vi "FetchSpecificationDataFromDb.vi"() -> ()   [LabVIEW 2019]
uses:
  <vilib>/addons/database/Auxilliary.llb/DB Tools Parameter Info.ctl
  <vilib>/addons/database/Auxilliary.llb/DB Tools DataTypes.ctl
  <vilib>/addons/database/Auxilliary.llb/DB Tools Parameter Dir.ctl
  <vilib>/addons/database/Auxilliary.llb/DB Tools Format Datetime String (Time Stamp).vi
  <vilib>/addons/database/Connection.llb/DB Tools Open Connec (String).vi
  <vilib>/addons/database/Command.llb/Cmd Set Parameter Value (C).vi
  <vilib>/addons/database/Command.llb/Cmd Execute.vi
  <vilib>/addons/database/Recordset.llb/Rec Fetch Recordset Data (CR).vi
  <vilib>/addons/database/Recordset.llb/Rec Destroy - Command.vi
  <vilib>/addons/database/Command.llb/Cmd Delete.vi
  <vilib>/addons/database/Recordset.llb/Rec Fetch String Data (CR).vi
  <vilib>/addons/database/NI_Database_API.lvlib
panel:
  out "tables":string[](array[string])
  out "data":string
  out "Program end (seconds)":dbl
  out "Programe fetched data time":timestamp
  out "Programme start time":timestamp
  out "size(s)":i32[](array[numeric])
  in  "Provide your To DateTime here":timestamp
  in  "Provide your from  DateTime here":timestamp
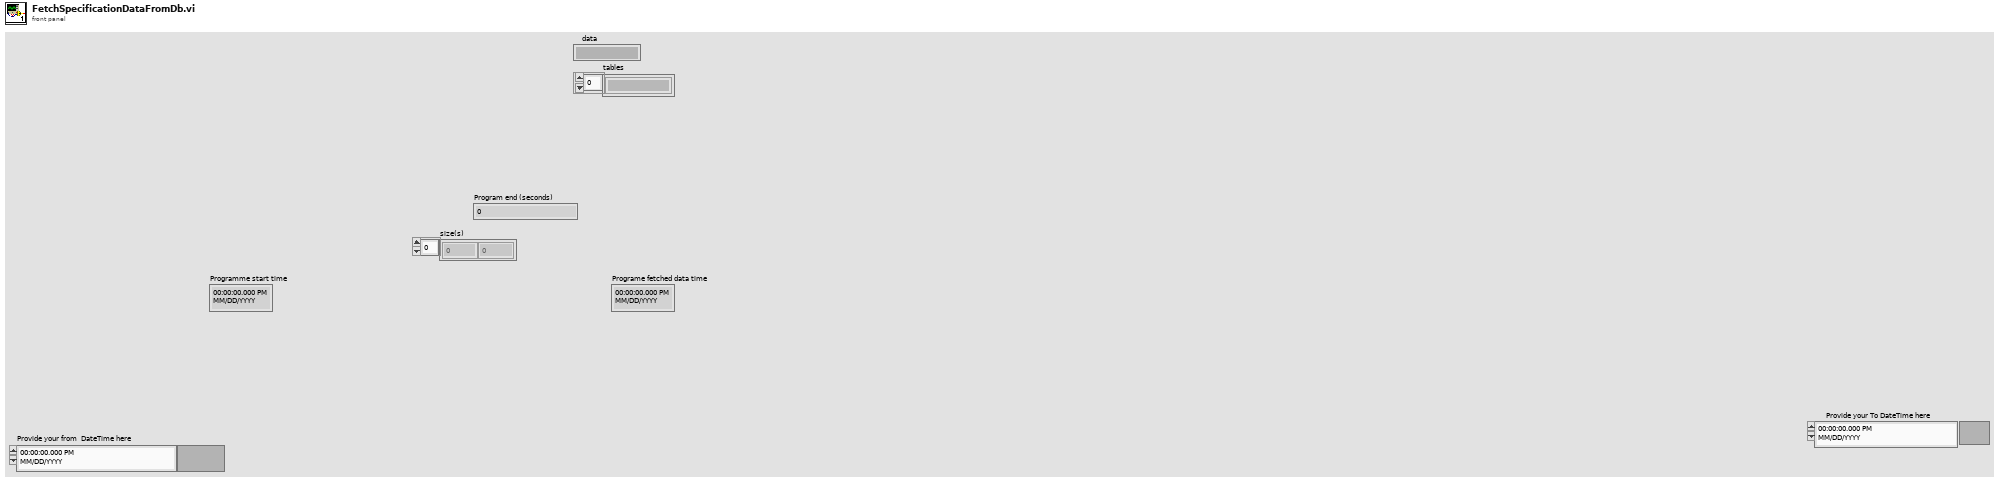
[diagram p1: front panel]
types:
  T1 = typedef "NI_Database_API.lvlib/DB Tools Parameter Info.ctl" = cluster{"parameter name":string, "type":T2, "direction":T3, "value":variant}
  T2 = typedef "NI_Database_API.lvlib/DB Tools DataTypes.ctl" = enum16{"String", "Long (I32)", "Single (SGL)", "Double (DBL)", "Date/Time", "Binary"}
  T3 = typedef "NI_Database_API.lvlib/DB Tools Parameter Dir.ctl" = enum32{"Input", "Output", "Input/Output", "Return Value"}
  T4 = typedef "NI_Database_API.lvlib/Conn ObjectReference.ctl" = refnum<k1>
  T5 = typedef "NI_Database_API.lvlib/Cmd ObjectReference.ctl" = refnum<k1>
  T6 = typedef "NI_Database_API.lvlib/Cmd-Rec Object Reference.ctl" = refnum<k1>
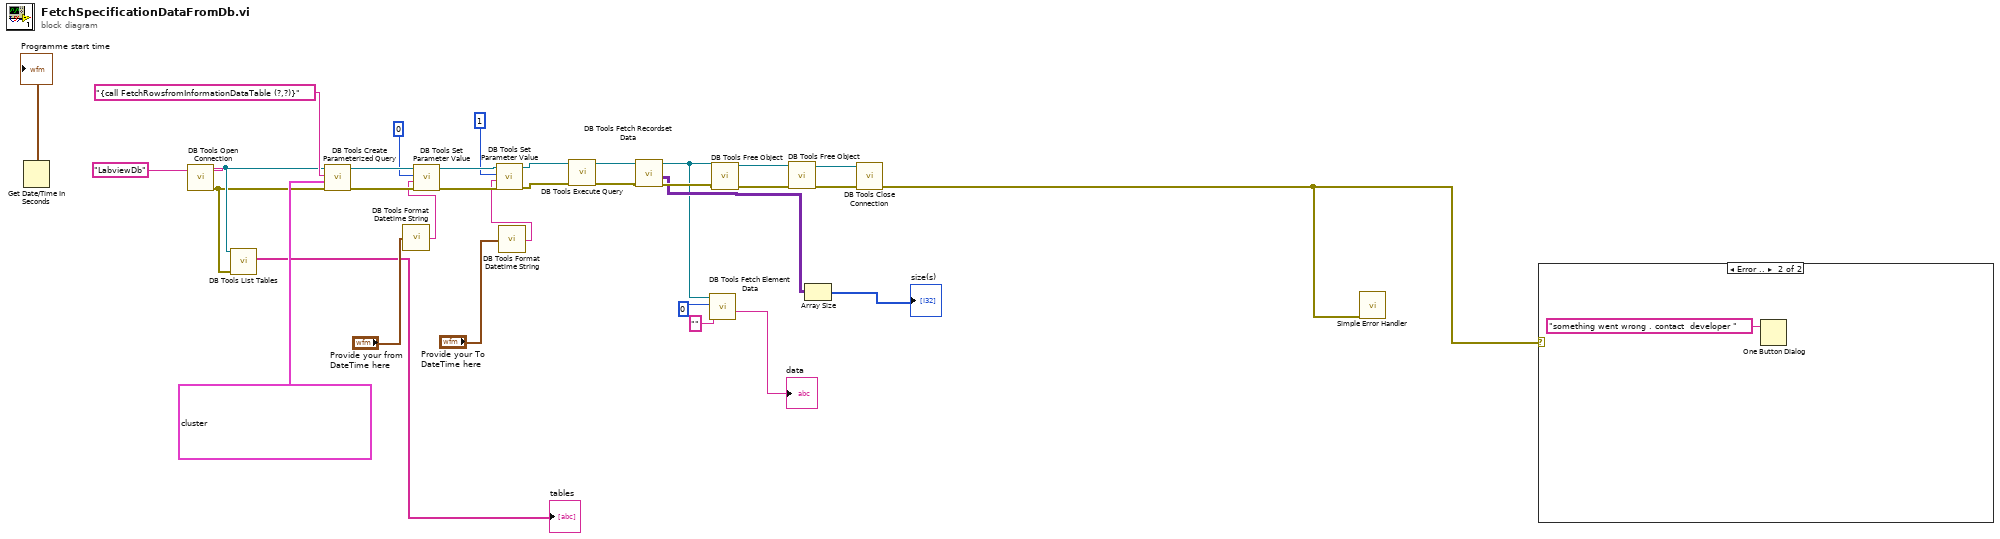
[diagram p0: block diagram]
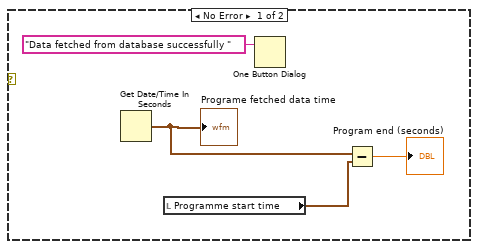
[diagram p2: hidden frame]
diagram:
  n1 = Get Date/Time In Seconds() -> (seconds since 1Jan1904=→"Programme start time":timestamp)
  n2 = call-poly <vilib>:"DB Tools Open Connection.vi"("connection information"="LabviewDb") -> ("error out"=w2:errorcluster, "connection reference"=w3:T4)  [unwired: 7 in]
  n3 = call <vilib>:"DB Tools List Tables.vi"("error in (no error)"=w2, "connection reference"=w3) -> ("tables"=→"tables":string[])  [unwired: 3 in, 2 out]
  n4 = call <vilib>:"DB Tools Create Parameterized Query.vi"("error in (no error)"=w2, "parameters"=T1[] [{"parameter name"="fromDate", "type"=enum."Date/Time", "direction"=enum."Input", "value"=variant}, {"parameter name"="toDate", "type"=enum."Date/Time", "direction"=enum."Input", "value"=variant}], "SQL query"="{call FetchRowsfromInformationDataTable (?,?)}", "connection reference"=w3) -> ("error out"=w30:errorcluster, "command reference"=w29:T5)  [unwired: 3 in, 1 out]
  n5 = call-poly <vilib>:"DB Tools Format Datetime String.vi"("time stamp"="Provide your from  DateTime here") -> ("date/time string"=w16:string)
  n6 = call-poly <vilib>:"DB Tools Set Parameter Value.vi"("error in (no error)"=w30, "value"=w16, "parameter index"=0, "command reference"=w29) -> ("error out"=w27:errorcluster, "command reference out"=w26:T5)  [unwired: 4 in]
  n7 = call-poly <vilib>:"DB Tools Format Datetime String.vi"("time stamp"="Provide your To DateTime here") -> ("date/time string"=w14:string)
  n8 = call-poly <vilib>:"DB Tools Set Parameter Value.vi"("error in (no error)"=w27, "value"=w14, "parameter index"=1, "command reference"=w26) -> ("error out"=w23:errorcluster, "command reference out"=w24:T5)  [unwired: 4 in]
  n9 = call-poly <vilib>:"DB Tools Execute Query.vi"("error in (no error)"=w23, "command reference"=w24) -> ("error out"=w11:errorcluster, "command-recordset reference"=w12:T6)  [unwired: 6 in]
  n10 = call-poly <vilib>:"DB Tools Fetch Recordset Data.vi"("error in (no error)"=w11, "command-recordset reference"=w12) -> ("error out"=w22:errorcluster, "recordset data"=w8:variant[][], "command-recordset reference out"=w7:T6)  [unwired: 3 in]
  n11 = call-poly <vilib>:"DB Tools Fetch Element Data.vi"("type"="", "column index"=0, "command-recordset reference"=w7) -> ("data"=→"data":string)  [unwired: 4 in, 2 out]
  n12 = call-poly <vilib>:"DB Tools Free Object.vi"("error in (no error)"=w22, "command-recordset reference"=w7) -> ("error out"=w20:errorcluster, "command reference"=w21:T5)  [unwired: 8 in]
  n13 = call-poly <vilib>:"DB Tools Free Object.vi"("error in (no error)"=w20, "command reference"=w21) -> ("error out"=w18:errorcluster, "connection reference"=w19:T4)  [unwired: 8 in]
  n14 = Array Size(array=w8) -> (size(s)=→"size(s)":i32[])
  n15 = call <vilib>:"DB Tools Close Connection.vi"("error in (no error)"=w18, "connection reference"=w19) -> ("error out"=w13:errorcluster)  [unwired: 5 in]
  n16 = call <vilib>:"Simple Error Handler.vi"("error in (no error)"=w13) -> ()  [unwired: 4 in, 5 out]
  n17 = case shown="Error .." w13 {
    frame No Error {
      n18 = Get Date/Time In Seconds() -> (seconds since 1Jan1904=w35:timestamp)
      "Programe fetched data time" <- w35
      n19 = local read "Programme start time"() -> (w34:timestamp)
      n20 = One Button Dialog(message="Data fetched from database successfully ") -> ()  [unwired: 1 in, 1 out]
      n21 = Subtract(x=w35, y=w34) -> (x-y=→"Program end (seconds)":dbl)
    }
    frame Error {
      n22 = One Button Dialog(message="something went wrong . contact  developer ") -> ()  [unwired: 1 in, 1 out]
    }
  }
